vi "Day 08 pt b.vi"() -> ()   [LabVIEW 2020]
uses:
  tree--cluster.ctl
panel:
  out "max value":i32
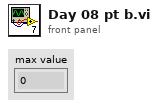
[diagram p1: front panel]
types:
  T1 = typedef "tree--cluster.ctl" = cluster{"Visible":bool, "Height":i32, "View up":i32, "View down":i32, "View left":i32, "View right":i32, "ViewTotal":i32}
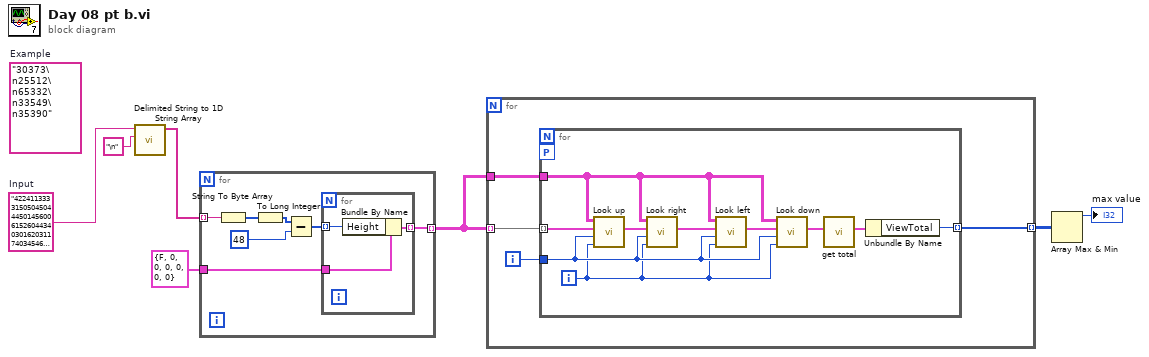
[diagram p0: block diagram]
diagram:
  w2 = "422411333315050450444501456006152604434030162031174034546313212413064150120521030152355534203000121\n301324204451515335252342253126503010214314026675523135330307170405066545120014006214521335013332134\n410011302103513543254453460342420630261341511764171765703774273674310415535166643155002215230224343\n103430412453541534313620414103230457371320115213510406561165762764547335046351220043205123531400041\n431144033221543442550410360065613506340166441027415155772664554705330520251311025141223233351402243\n213325510034542655030015455216430162202777001070241326522045362063054665216550230550303504355415521\n..."  # Input
  (unwired) "30373\n25512\n65332\n33549\n35390"  # Example
  n1 = call <vilib>:"Delimited String to 1D String Array.vi"("delimiter"="\n", "delimited string"=w2) -> ("string array"=w6:string[])  [unwired: 9 in]
  n2 = for {
    tunnel: w6 -> [w14] mode=indexing
    tunnel: [w8] -> w1 mode=indexing
    tunnel: T1 {"Visible"=FALSE, "Height"=0, "View up"=0, "View down"=0, "View left"=0, "View right"=0, "ViewTotal"=0} ("Tree") -> [w9]
    n3 = String To Byte Array(string=w14) -> (unsigned byte array=w13:u8[])
    n4 = To Long Integer(number=w13) -> (32bit integer=w11:i32[])
    n5 = Subtract(x=w11, y=48) -> (x-y=w10:i32[])
    n6 = for {
      tunnel: w10 -> [w16] mode=indexing
      tunnel: w9 -> [w17]
      tunnel: [w15] -> w8 mode=indexing
      n7 = Bundle By Name(cluster=w17, "Height"=w16) -> (w15:T1)
    }
  }
  n8 = for {
    tunnel: w1 -> [w21] mode=indexing
    tunnel: [w19] -> w4 mode=indexing
    tunnel: w1 -> [w18]
    i -> [w20]
    n9 = for {
      tunnel: w21 -> [w31] mode=indexing
      tunnel: w20 -> [w26]
      tunnel: [w23] -> w19 mode=indexing
      tunnel: w18 -> [w22]
      workers-P: _ -> [_]
      i -> [w25]
      n10 = call "Look up.vi"("column"=w25, "row"=w26, "Tree"=w31, "Array"=w22) -> ("output cluster"=w30:T1)  [unwired: 7 in]
      n11 = call "Look right.vi"("column"=w25, "row"=w26, "Tree"=w30, "Array"=w22) -> ("output cluster"=w29:T1)  [unwired: 7 in]
      n12 = call "Look left.vi"("column"=w25, "row"=w26, "Tree"=w29, "Array"=w22) -> ("output cluster"=w28:T1)  [unwired: 7 in]
      n13 = call "Look down.vi"("column"=w25, "row"=w26, "Tree"=w28, "Array"=w22) -> ("output cluster"=w27:T1)  [unwired: 7 in]
      n14 = call "get total.vi"("Tree"=w27) -> ("Tree 2"=w24:T1)  [unwired: 10 in]
      n15 = Unbundle By Name(w24) -> ("ViewTotal"=w23:i32)
    }
  }
  n16 = Array Max & Min(array=w4) -> (max value=→"max value":i32)  [unwired: 3 out]
